vi "Read Shared Variables - SuNLaMP AI - Hot.vi"(9 "channel errors in (no errors)":errorcluster[](array[cluster])) -> (1 "channel errors out":errorcluster[](array[cluster]), 2 "data":dbl[](array[numeric]), 3 "UUIDs":string[](array[string])=["Flow Rate [g/s]", "Density [g/cm^3]", "Return Filter dP [psid]", "Outlet Filter and Flowmeter dp [psid]", "Cooler dP [psid]", "Cooler CO2 In [F]", "Cooler CO2 Out [F]", "Pump Frequency [%]", "Recirc Valve Open [%]"])   [LabVIEW 2020]
uses:
  <vilib>/Utility/error.llb/Error Cluster From Error Code.vi
  <vilib>/ErrorRing/Error Ring.xnode
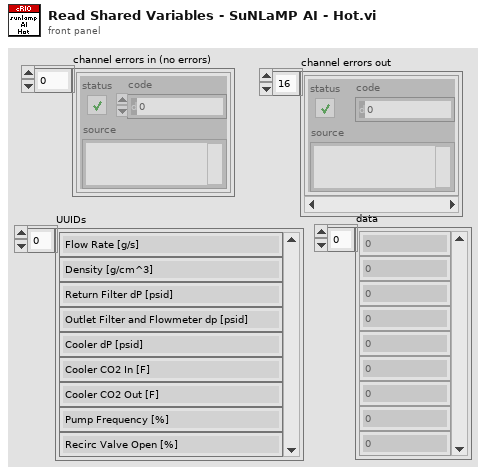
[diagram p1: front panel]
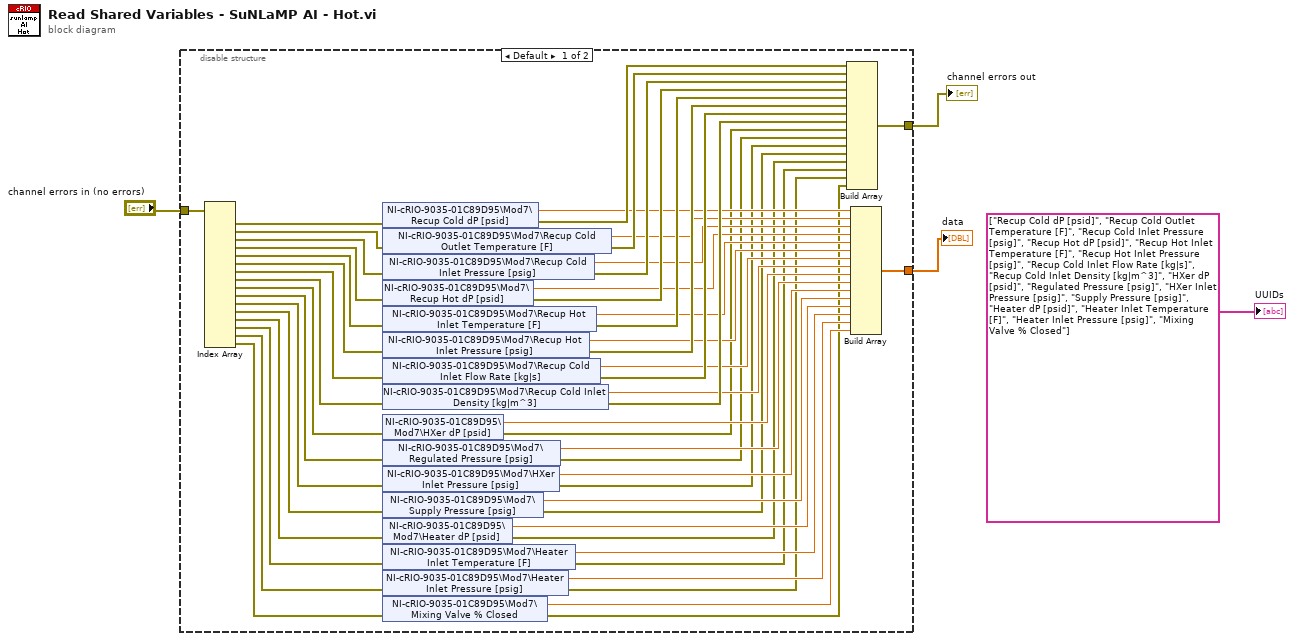
[diagram p0: block diagram]
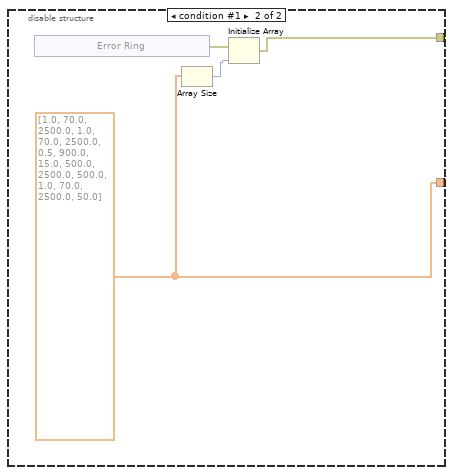
[diagram p2: hidden frame]
diagram:
  n1 = disable-structure shown="Default" {
    disable-tunnel: [w39 w56] -> w4
    disable-tunnel: [w38 w57] -> w2
    disable-tunnel: "channel errors in (no errors)" -> [w37 _]
    frame condition #0 (active) {
      n2 = Index Array(array=w37) -> (element #1=w36:errorcluster, element #2=w35:errorcluster, element #3=w34:errorcluster, element #4=w33:errorcluster, element #5=w32:errorcluster, element #6=w31:errorcluster, element #7=w30:errorcluster, element #8=w29:errorcluster, element #9=w28:errorcluster, element #10=w27:errorcluster, element #11=w26:errorcluster, element #12=w25:errorcluster, element #13=w24:errorcluster, element #14=w23:errorcluster, element #15=w22:errorcluster, element #16=w21:errorcluster)  [unwired: 16 in]
      n3 = shared-variable "NI-cRIO-9035-01C89D95\\Mod7\\Recup Cold dP [psid]"(error in=w36) -> (w40:dbl, error out=w48:errorcluster)
      n4 = shared-variable "NI-cRIO-9035-01C89D95\\Mod7\\Recup Cold Outlet Temperature [F]"(error in=w35) -> (w41:dbl, error out=w49:errorcluster)
      n5 = shared-variable "NI-cRIO-9035-01C89D95\\Mod7\\Recup Cold Inlet Pressure [psig]"(error in=w34) -> (w42:dbl, error out=w50:errorcluster)
      n6 = shared-variable "NI-cRIO-9035-01C89D95\\Mod7\\Recup Hot dP [psid]"(error in=w33) -> (w43:dbl, error out=w51:errorcluster)
      n7 = shared-variable "NI-cRIO-9035-01C89D95\\Mod7\\Recup Hot Inlet Temperature [F]"(error in=w32) -> (w44:dbl, error out=w52:errorcluster)
      n8 = shared-variable "NI-cRIO-9035-01C89D95\\Mod7\\Recup Hot Inlet Pressure [psig]"(error in=w31) -> (w45:dbl, error out=w53:errorcluster)
      n9 = shared-variable "NI-cRIO-9035-01C89D95\\Mod7\\Recup Cold Inlet Flow Rate [kg|s]"(error in=w30) -> (w46:dbl, error out=w54:errorcluster)
      n10 = shared-variable "NI-cRIO-9035-01C89D95\\Mod7\\Recup Cold Inlet Density [kg|m^3]"(error in=w29) -> (w47:dbl, error out=w55:errorcluster)
      n11 = shared-variable "NI-cRIO-9035-01C89D95\\Mod7\\HXer dP [psid]"(error in=w28) -> (w20:dbl, error out=w12:errorcluster)
      n12 = shared-variable "NI-cRIO-9035-01C89D95\\Mod7\\Regulated Pressure [psig]"(error in=w27) -> (w19:dbl, error out=w11:errorcluster)
      n13 = shared-variable "NI-cRIO-9035-01C89D95\\Mod7\\HXer Inlet Pressure [psig]"(error in=w26) -> (w18:dbl, error out=w10:errorcluster)
      n14 = shared-variable "NI-cRIO-9035-01C89D95\\Mod7\\Supply Pressure [psig]"(error in=w25) -> (w17:dbl, error out=w9:errorcluster)
      n15 = shared-variable "NI-cRIO-9035-01C89D95\\Mod7\\Heater dP [psid]"(error in=w24) -> (w16:dbl, error out=w8:errorcluster)
      n16 = shared-variable "NI-cRIO-9035-01C89D95\\Mod7\\Heater Inlet Temperature [F]"(error in=w23) -> (w15:dbl, error out=w7:errorcluster)
      n17 = shared-variable "NI-cRIO-9035-01C89D95\\Mod7\\Heater Inlet Pressure [psig]"(error in=w22) -> (w14:dbl, error out=w6:errorcluster)
      n18 = shared-variable "NI-cRIO-9035-01C89D95\\Mod7\\Mixing Valve % Closed"(error in=w21) -> (w13:dbl, error out=w5:errorcluster)
      n19 = Build Array(w48, w49, w50, w51, w52, w53, w54, w55, w12, w11, w10, w9, w8, w7, w6, w5) -> (w38:errorcluster[])
      n20 = Build Array(w40, w41, w42, w43, w44, w45, w46, w47, w20, w19, w18, w17, w16, w15, w14, w13) -> (w39:dbl[])
    }
    frame condition #1 {
      w56 = dbl[] [1.0, 70.0, 2500.0, 1.0, 70.0, 2500.0, 0.5, 900.0, 15.0, 500.0, 2500.0, 500.0, 1.0, 70.0, 2500.0, 50.0] ("data")
      n21 = xnode "Error Ring"() -> ("error out"=w59:errorcluster)
      n22 = Array Size(array=w56) -> (size(s)=w58:i32)
      n23 = Initialize Array(w59, w58) -> (w57:errorcluster[])
    }
  }
  "data" <- w4
  "channel errors out" <- w2
  "UUIDs" <- string[] ["Recup Cold dP [psid]", "Recup Cold Outlet Temperature [F]", "Recup Cold Inlet Pressure [psig]", "Recup Hot dP [psid]", "Recup Hot Inlet Temperature [F]", "Recup Hot Inlet Pressure [psig]", "Recup Cold Inlet Flow Rate [kg|s]", "Recup Cold Inlet Density [kg|m^3]", "HXer dP [psid]", "Regulated Pressure [psig]", "HXer Inlet Pressure [psig]", "Supply Pressure [psig]", "Heater dP [psid]", "Heater Inlet Temperature [F]", "Heater Inlet Pressure [psig]", "Mixing Valve % Closed"]
